vi "Stream_raw_data.vi"(8 "error in":errorcluster, 10 "Data flow controls":T1, 11 "VISA resource name in":refnum<visa-resource-name>) -> (0 "error out":errorcluster, 1 "Timestamp":timestamp, 2 "Data flow controls out":T1, 3 "VISA resource name out":refnum<visa-resource-name>, 5 "Read buffer":string)   [LabVIEW 2016]
uses:
  <vilib>/Instr/_visa.llb/VISA Flush IO Buffer Mask.ctl
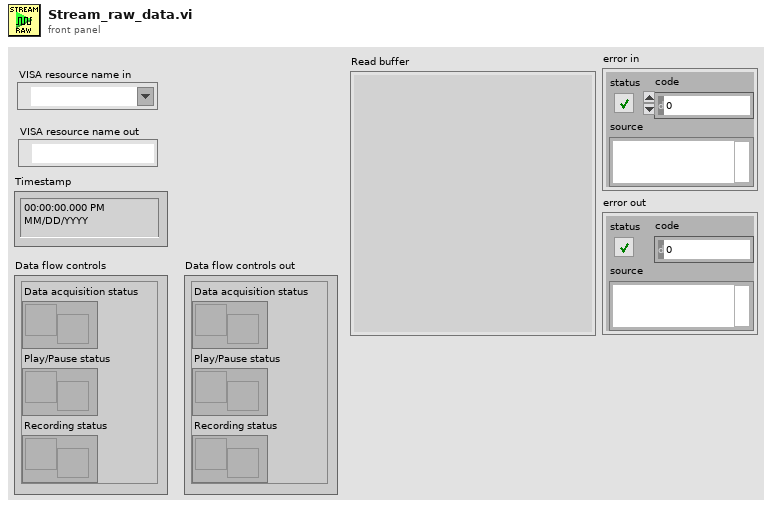
[diagram p1: front panel]
types:
  T1 = cluster{"Data acquisition status":refnum<notifier>, "Play/Pause status":refnum<notifier>, "Recording status":refnum<notifier>}
  T2 = typedef "VISA Flush IO Buffer Mask.ctl" = u16
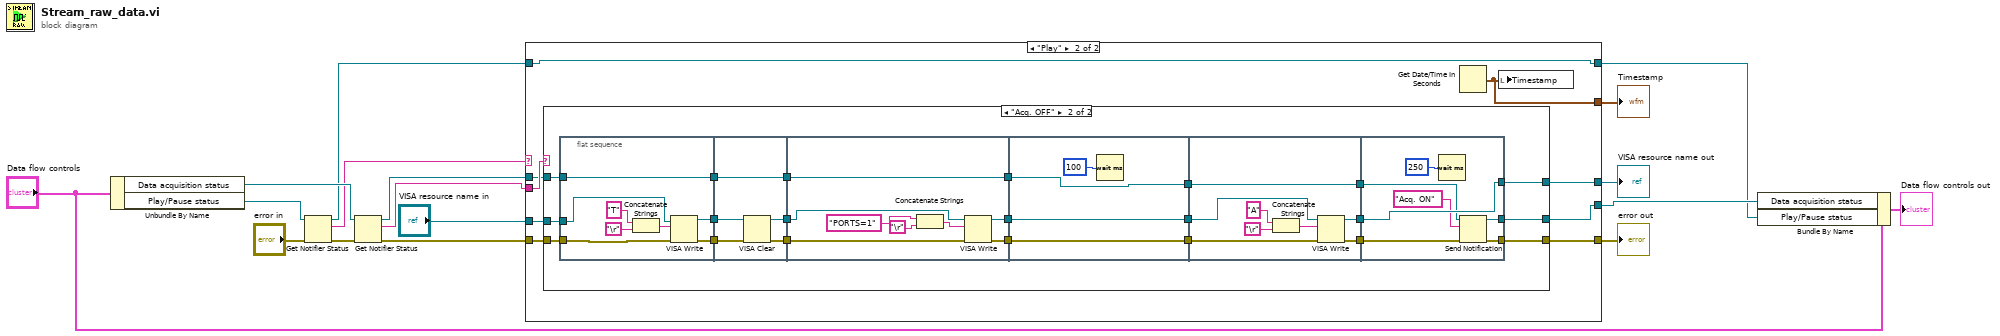
[diagram p0: block diagram]
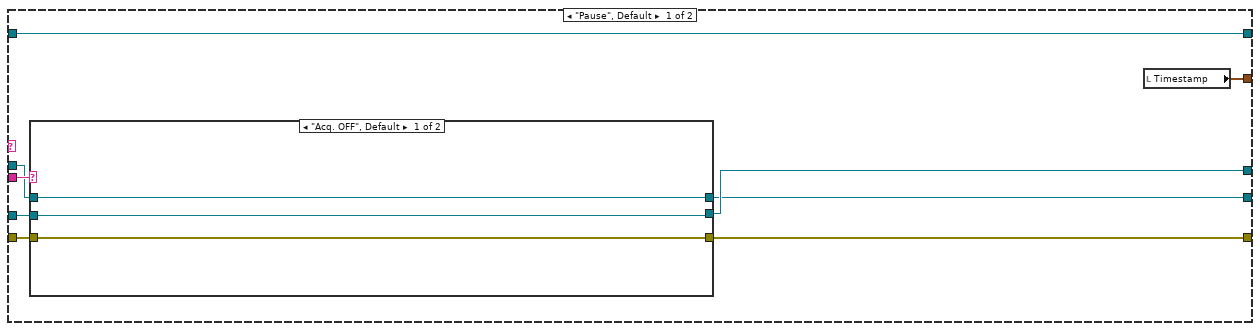
[diagram p2: hidden frame]
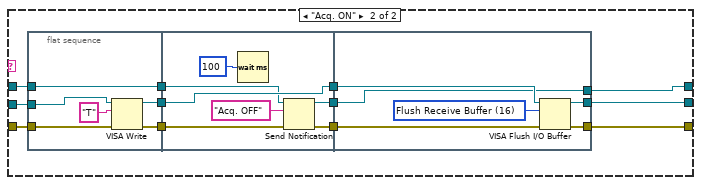
[diagram p3: hidden frame]
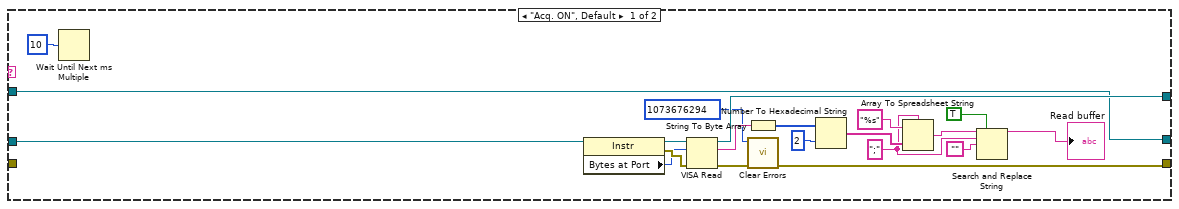
[diagram p4: hidden frame]
diagram:
  n1 = Unbundle By Name("Data flow controls") -> ("Data acquisition status"=w15:refnum<notifier>, "Play/Pause status"=w14:refnum<notifier>)
  n2 = Get Notifier Status(notifier=w14, error in (no error)="error in") -> (notifier out=w9:refnum<notifier>, current notification=w13:string, error out=w10:errorcluster)  [unwired: 2 out]
  n3 = Get Notifier Status(notifier=w15, error in (no error)=w10) -> (notifier out=w8:refnum<notifier>, current notification=w12:string, error out=w3:errorcluster)  [unwired: 2 out]
  n4 = case shown="\"Play\"" w13 {
    tunnel: [w25 w68] -> w16
    tunnel: "VISA resource name in" -> [w26 w69]
    tunnel: w12 -> [w24 w65]
    tunnel: w9 -> [w21 w62]
    tunnel: w8 -> [w23 w64]
    tunnel: [w22 w63] -> w6
    tunnel: [w21 w62] -> w5
    tunnel: w3 -> [w20 w67]
    tunnel: [w19 w66] -> w2
    tunnel: [w18 w61] -> w1
    frame "Pause", Default {
      n5 = case shown="\"Acq. OFF\", Default" w24 {
        tunnel: w26 -> [w29 w39]
        tunnel: [w29 w38] -> w25
        tunnel: w23 -> [w28 w32]
        tunnel: [w28 w31] -> w22
        tunnel: w20 -> [w27 w35]
        tunnel: [w27 w34] -> w19
        frame "Acq. OFF", Default {
        }
        frame "Acq. ON" {
          n6 = flat-sequence {
            tunnel: w39 -> [w47]
            tunnel: [w46] -> w41
            tunnel: [w45] -> w40
            tunnel: w35 -> [w43]
            tunnel: [w42] -> w33
            tunnel: w32 -> [w42]
            tunnel: w41 -> [w53]
            tunnel: w40 -> [w52]
            tunnel: [w53] -> w37
            tunnel: [w51] -> w36
            tunnel: w33 -> [w49]
            tunnel: [w48] -> w30
            tunnel: [w58] -> w38
            tunnel: w37 -> [w59]
            tunnel: w36 -> [w60]
            tunnel: [w56] -> w34
            tunnel: [w55] -> w31
            tunnel: w30 -> [w55]
            frame #0 {
              n7 = VISA Write(VISA resource name=w47, write buffer="T", error in (no error)=w43) -> (VISA resource name out=w46:refnum<visa-resource-name>, error out=w45:errorcluster)  [unwired: 1 out]
            }
            frame #1 {
              n8 = Wait (ms)(milliseconds to wait=u32 100) -> ()  [unwired: 1 out]
              n9 = Send Notification(notification="Acq. OFF", notifier=w49, error in (no error)=w52) -> (notifier out=w48:refnum<notifier>, error out=w51:errorcluster)
            }
            frame #2 {
              w57 = T2 16 items=["Flush Receive Buffer"=16, "Write Transmit Buffer to Device"=32, "Flush Receive Buffer (No I/O)"=64, "Flush Transmit Buffer"=128] ("Mask")
              n10 = VISA Flush I/O Buffer(VISA resource name=w59, mask (16)=w57, error in (no error)=w60) -> (VISA resource name out=w58:refnum<visa-resource-name>, error out=w56:errorcluster)
            }
          }
        }
      }
      n11 = local read "Timestamp"() -> (w18:timestamp)
    }
    frame "Play" {
      n12 = case shown="\"Acq. OFF\"" w65 {
        tunnel: w69 -> [w89 w108]
        tunnel: [w85 w107] -> w68
        tunnel: [w72 w106] -> w66
        tunnel: w67 -> [_ w97]
        tunnel: w64 -> [w70 w91]
        tunnel: [w70 w90] -> w63
        frame "Acq. ON", Default {
          w79 = ";" ("delimiter (Tab)")
          n13 = Wait Until Next ms Multiple(millisecond multiple=u32 10) -> ()  [unwired: 1 out]
          n14 = property class="Instr"(reference=w89) -> (reference out=w88:refnum<visa-resource-name>, error out=w87:errorcluster, "Bytes at Port"=w86:u32)  [unwired: 1 in]
          n15 = VISA Read(VISA resource name=w88, byte count=w86, error in (no error)=w87) -> (VISA resource name out=w85:refnum<visa-resource-name>, read buffer=w77:string, error out=w73:errorcluster)  [unwired: 1 out]
          n16 = String To Byte Array(string=w77) -> (unsigned byte array=w84:u8[])
          n17 = call <vilib>:"Clear Errors.vi"("error in (no error)"=w73, "specific error code to clear (0: all)"=1073676294) -> ("error out"=w72:errorcluster)  [unwired: 4 in, 1 out]
          n18 = Number To Hexadecimal String(1:i16 2 ("width (-)"), 2:w84) -> (0:w82:string[])
          n19 = Array To Spreadsheet String(delimiter (Tab)=w79, array=w82, 3:"%s" ("format string")) -> (spreadsheet string=w80:string)
          n20 = Search and Replace String(replace all?=TRUE ("replace all? (F)"), input string=w80, search string=w79, replace string="") -> (result string=→"Read buffer":string)  [unwired: 4 in, 3 out]
        }
        frame "Acq. OFF" {
          n21 = flat-sequence {
            tunnel: w108 -> [w117]
            tunnel: [w118] -> w105
            tunnel: [w116] -> w104
            tunnel: w97 -> [w112]
            tunnel: [w111] -> w92
            tunnel: w91 -> [w111]
            tunnel: [w123] -> w99
            tunnel: [w122] -> w98
            tunnel: w104 -> [w121]
            tunnel: w105 -> [w120]
            tunnel: [w119] -> w93
            tunnel: w92 -> [w119]
            tunnel: w99 -> [w129]
            tunnel: [w128] -> w103
            tunnel: w98 -> [w127]
            tunnel: [w126] -> w102
            tunnel: [w124] -> w94
            tunnel: w93 -> [w124]
            tunnel: [w135] -> w101
            tunnel: [w134] -> w100
            tunnel: w102 -> [w134]
            tunnel: w103 -> [w135]
            tunnel: [w132] -> w95
            tunnel: w94 -> [w132]
            tunnel: [w138] -> w110
            tunnel: [w137] -> w109
            tunnel: w101 -> [w140]
            tunnel: w100 -> [w139]
            tunnel: [w136] -> w96
            tunnel: w95 -> [w136]
            tunnel: [w147] -> w106
            tunnel: w110 -> [w148]
            tunnel: w109 -> [w149]
            tunnel: [w149] -> w107
            tunnel: w96 -> [w146]
            tunnel: [w145] -> w90
            frame #0 {
              n22 = Concatenate Strings("T" ("write buffer"), "\r") -> (w113:string)
              n23 = VISA Write(VISA resource name=w117, write buffer=w113, error in (no error)=w112) -> (VISA resource name out=w118:refnum<visa-resource-name>, error out=w116:errorcluster)  [unwired: 1 out]
            }
            frame #1 {
              n24 = VISA Clear(VISA resource name=w120, error in (no error)=w121) -> (VISA resource name out=w123:refnum<visa-resource-name>, error out=w122:errorcluster)
            }
            frame #2 {
              n25 = Concatenate Strings("PORTS=1" ("write buffer"), "\r") -> (w130:string)
              n26 = VISA Write(VISA resource name=w129, write buffer=w130, error in (no error)=w127) -> (VISA resource name out=w128:refnum<visa-resource-name>, error out=w126:errorcluster)  [unwired: 1 out]
            }
            frame #3 {
              n27 = Wait (ms)(milliseconds to wait=u32 100) -> ()  [unwired: 1 out]
            }
            frame #4 {
              n28 = Concatenate Strings("A" ("write buffer"), "\r") -> (w141:string)
              n29 = VISA Write(VISA resource name=w140, write buffer=w141, error in (no error)=w139) -> (VISA resource name out=w137:refnum<visa-resource-name>, error out=w138:errorcluster)  [unwired: 1 out]
            }
            frame #5 {
              n30 = Wait (ms)(milliseconds to wait=u32 250) -> ()  [unwired: 1 out]
              n31 = Send Notification(notification="Acq. ON", notifier=w146, error in (no error)=w148) -> (notifier out=w145:refnum<notifier>, error out=w147:errorcluster)
            }
          }
        }
      }
      n32 = Get Date/Time In Seconds ("Current time")() -> (seconds since 1Jan1904=w61:timestamp)
      n33 = local write "Timestamp"(w61) -> ()
    }
  }
  "VISA resource name out" <- w16
  "error out" <- w2
  "Timestamp" <- w1
  n34 = Bundle By Name(cluster="Data flow controls", "Data acquisition status"=w6, "Play/Pause status"=w5) -> (→"Data flow controls out":T1)
